vi "Load Config.vi"(6 "Constants":refnum<class "Sequence Constants.lvclass">, 8 "error in (no error)":refnum<class "MultiErrors.lvclass">, 10 "Config Element":refnum<class "Config Element.lvclass">, 11 "Event Command Config in":refnum<class "Event Command Config.lvclass">) -> (0 "error out":refnum<class "MultiErrors.lvclass">, 3 "Event Command Config out":refnum<class "Event Command Config.lvclass">)   [LabVIEW 2020, in "VolatusSeqConfig.lvlib" / "Event Command Config.lvclass"]
uses:
  Event Command Config.lvclass
  VolatusErrorUtilities/MultiErrors/MultiErrors.lvclass
  lv-cdm/CDM-Config/Config Element/Config Element.lvclass
  Event Command Config.lvclass/Event Command Config.ctl
  Sequence Constants/Sequence Constants.lvclass
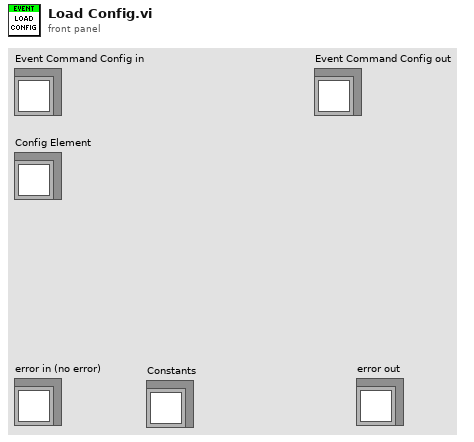
[diagram p1: front panel]
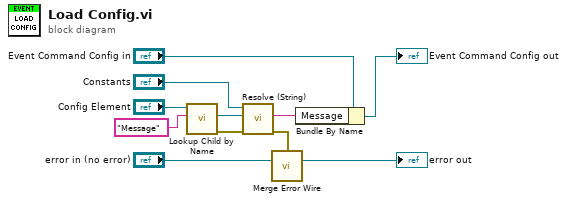
[diagram p0: block diagram]
diagram:
  n1 = call "Lookup Child by Name.vi"("Name"="Message", "Config Element in"="Config Element") -> ("error out"=w4:errorcluster, "Child"=w5:refnum<class "Config Element.lvclass">)  [unwired: 6 in, 2 out]
  n2 = call "Resolve (String).vi"("error in (no error)"=w4, "Element"=w5, "Sequence Constants in"="Constants") -> ("error out"=w1:errorcluster, "String Value"=w2:string)  [unwired: 6 in, 1 out]
  n3 = call "Merge Error Wire.vi"("error in (no error)"=w1, "MultiErrors in"="error in (no error)") -> ("MultiErrors out"=→"error out":refnum<class "MultiErrors.lvclass">)  [unwired: 13 in]
  n4 = Bundle By Name(cluster="Event Command Config in", "Message"=w2) -> (→"Event Command Config out":refnum<class "Event Command Config.lvclass">)
